vi "convert WFS array 1D to 2D.vi"(9 "spots_y":i32, 10 "spots_x":i32, 11 "WF 1D input":sgl[](array[numeric])) -> (3 "FW 2D output":sgl[][](array[numeric]))   [LabVIEW 2016]
doc: "Convert 1D array of WFS data into 2D array"
panel:
  # "Convert 1D array of WFS data into 2D array"
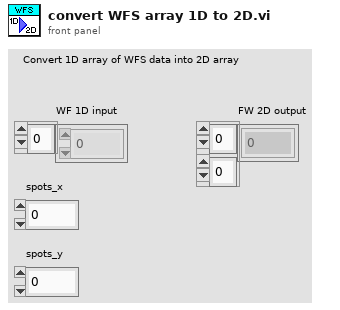
[diagram p1: front panel]
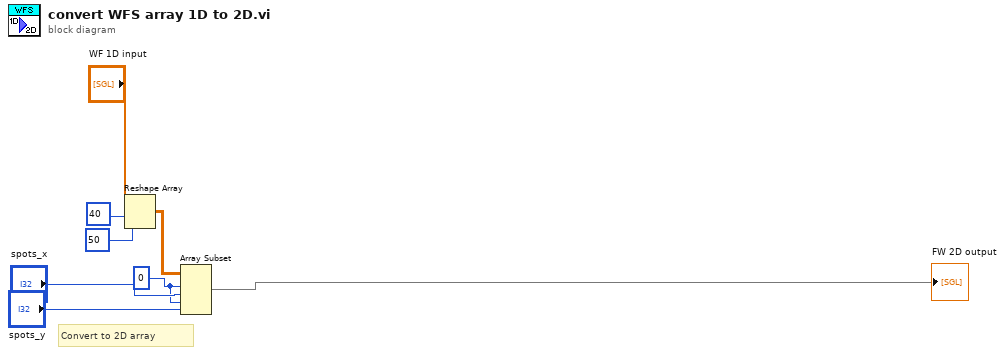
[diagram p0: block diagram]
diagram:
  w5 = 0 ("index")
  # "Convert to 2D array"
  n1 = Reshape Array("WF 1D input", 40 ("dimension size"), 50 ("dimension size")) -> (w4:sgl[][])
  n2 = Array Subset(array=w4, index (row)=w5, length (row)="spots_x", index (col)=w5, length (col)="spots_y") -> (→"FW 2D output":sgl[][])
